vi "WaitForCommStartStop.vi"(8 "error in (no error)":errorcluster, 11 "VISA Refnum in":refnum<visa-resource-name>) -> (0 "error out":errorcluster, 1 "timeout":bool, 2 "Bytes at Port":u32, 3 "VISA Refnum out":refnum<visa-resource-name>, 4 "Msecs to stopped":u32, 5 "Msecs to first byte":u32)   [LabVIEW 2013]
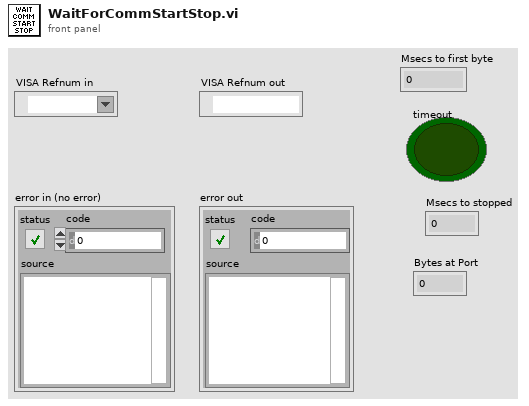
[diagram p1: front panel]
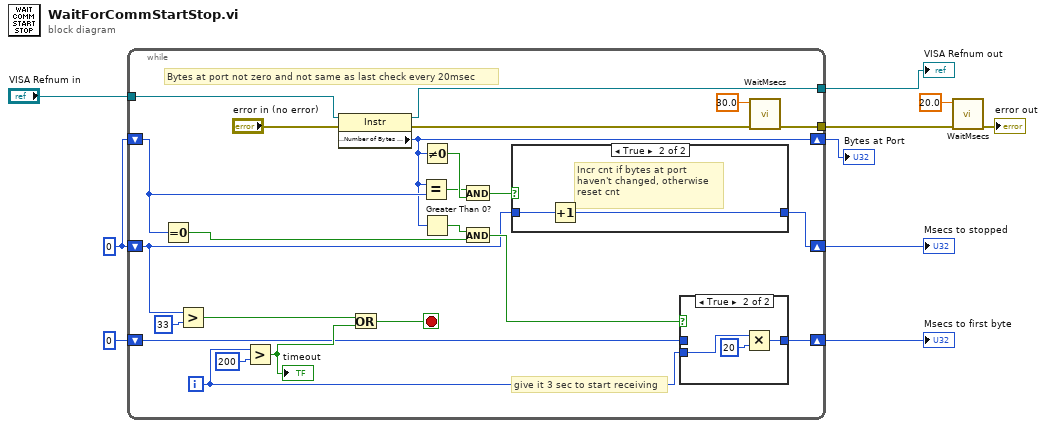
[diagram p0: block diagram]
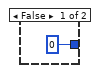
[diagram p3: hidden frame]
diagram:
  w4 = u32 0 ("Bytes at Port")
  n1 = while {
    tunnel: [w32] -> w8
    shift-right: [w20] -> w10
    shift-left: w4 -> [w21]
    tunnel: "VISA Refnum in" -> [w25]
    tunnel: [w24] -> w5
    shift-right: [w22] -> w1
    shift-left: w4 -> [w13]
    shift-right: [w15] -> w2
    shift-left: u32 0 ("Bytes at Port") -> [w16]
    i -> [w14]
    stop <- w28 stop-if-true
    # "give it 3 sec to start receiving"
    # "Bytes at port not zero and not same as last check every 20msec"
    n2 = Equal To 0?(x=w21) -> (x = 0?=w18:bool)
    n3 = Greater?(x=w13, y=u32 33) -> (0:w11:bool)
    n4 = Greater?(x=w14, y=200) -> (0:w27:bool)
    "timeout" <- w27
    n5 = property class="Instr"(reference=w25, error in="error in (no error)") -> (reference out=w24:refnum<visa-resource-name>, error out=w33:errorcluster, "Serial Settings:Number of Bytes at Serial Port"=w20:u32)
    n6 = Or(x=w11, y=w27) -> (x .or. y?=w28:bool)
    n7 = Equal?(x=w20, y=w21) -> (x = y?=w29:bool)
    n8 = Not Equal To 0?(x=w20) -> (x != 0?=w30:bool)
    n9 = Greater Than 0?(x=w20) -> (x > 0?=w17:bool)
    n10 = And(x=w29, y=w30) -> (x .and. y?=w23:bool)
    n11 = And(x=w17, y=w18) -> (x .and. y?=w19:bool)
    n12 = case shown="True" w23 {
      tunnel: w13 -> [_ w41]
      tunnel: [u32 0 w40] -> w22
      frame False {
      }
      frame True {
        # "Incr cnt if bytes at port\nhaven't changed, otherwise\nreset cnt"
        n13 = Increment(x=w41) -> (x+1=w40:u32)
      }
    }
    n14 = case shown="True" w19 {
      tunnel: w16 -> [w35 _]
      tunnel: [w35 w38] -> w15
      tunnel: w14 -> [_ w37]
      frame False {
      }
      frame True {
        n15 = Multiply(x=w37, y=20) -> (x*y=w38:i32)
      }
    }
    n16 = call "WaitMsecs.vi"("error in (no error)"=w33, "Wait Msecs"=30.0) -> ("error out"=w32:errorcluster)  [unwired: 9 in]
  }
  "Bytes at Port" <- w10
  "VISA Refnum out" <- w5
  "Msecs to first byte" <- w2
  "Msecs to stopped" <- w1
  n17 = call "WaitMsecs.vi"("error in (no error)"=w8, "Wait Msecs"=20.0) -> ("error out"=→"error out":errorcluster)  [unwired: 9 in]
